vi "Build Dialog.vi"(8 "error in (no error)":errorcluster, 10 "Dialog VI":refnum<vi>, 11 "CS++Actor in":refnum<class "CS++Actor.lvclass">) -> (0 "error out":errorcluster, 3 "CS++Actor out":refnum<class "CS++Actor.lvclass">)   [LabVIEW 2015, in "CS++Actor.lvlib" / "CS++Actor.lvclass"]
uses:
  CS++Actor.lvclass
  <vilib>/Utility/traverseref.llb/TRef TravTarget.ctl
  <vilib>/Utility/VariantDataType/Type.ctl
  CS++Actor.lvclass/CS++Actor.ctl
  <vilib>/Utility/VariantDataType/VariantType.lvlib
  <vilib>/Utility/traverseref.llb/VI Scripting - Traverse.lvlib
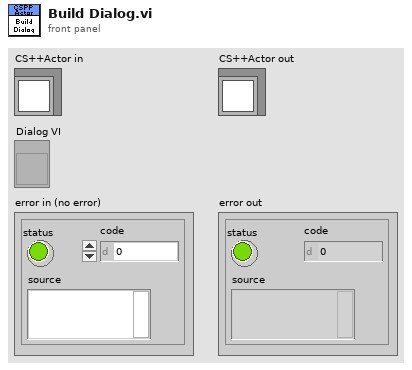
[diagram p1: front panel]
types:
  T1 = typedef "VariantType.lvlib/Type.ctl" = enum8{"Invalid Type", "Void", "I8", "I16", "I32", "I64", "U8", "U16", "U32", "U64", "Single Float", "Double Float", "Extended Float", "Single Complex", "Double Complex", "Extended Complex", "Enum U8", "Enum U16", "Enum U32", "Enum U64", "Single Float With Unit", "Double Float With Unit", "Extended Float With Unit", "Single Complex with Unit", "Double Complex with Unit", "Extended Complex with Unit", "Boolean", "String", "Path", "Picture", "Tag", "Array", "Cluster", "Variant", "LV Variant", "Waveform", "Timestamp", "Digital Waveform", "Digital Data", "ExpressData", "Refnum", "External Data", "VI", "Poly VI", "LabVIEW Class Instance", "Fixed Point"}
  T2 = typedef "TRef TravTarget.ctl" = enum16{"FP", "BD", "Other"}
  T3 = enum8{"Probe", "Diagram", "Panel Control", "3D Panel Control", "Dialog Panel Control", "Panel Indicator", "3D Panel Indicator", "Dialog Panel Indicator", "Power PC Control", "Power PC Indicator", "Silver Control", "Silver Indicator"}
  T4 = enum16{"Invalid Wire Rule", "Required", "Recommended", "Optional", "Dynamic Dispatch"}
  T5 = typedef "LVRectTypeDef.ctl" = cluster{"Left":i16, "Top":i16, "Right":i16, "Bottom":i16}
  T6 = enum16{"Invalid Wire Rule", "Required", "Recommended", "Optional", "Dynamic Dispatch"}[]
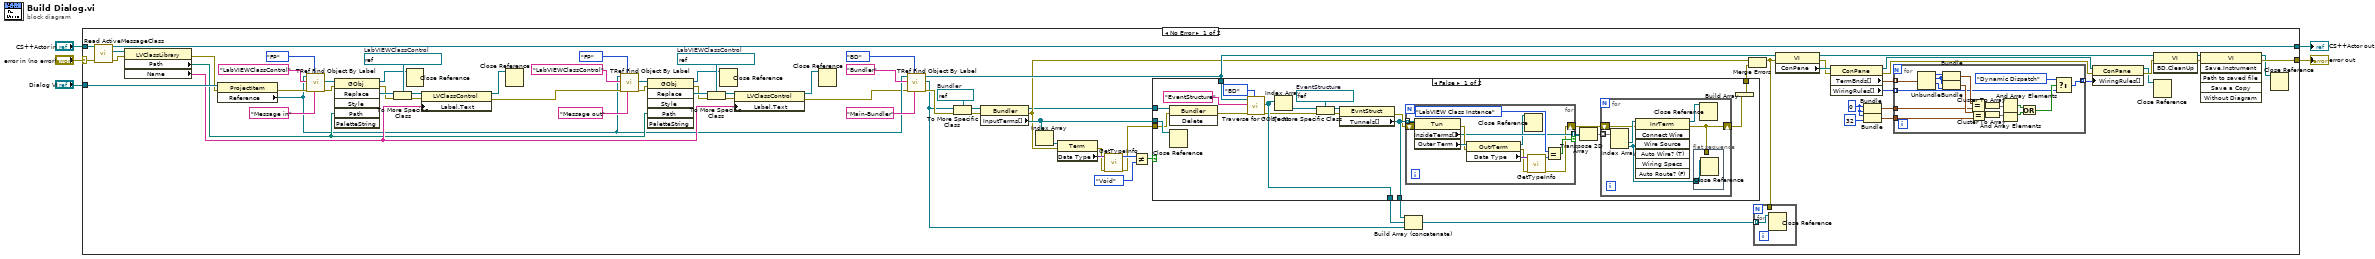
[diagram p0: block diagram]
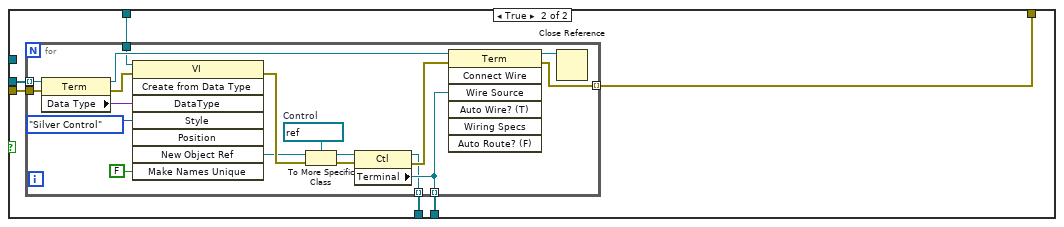
[diagram p2: hidden frame]
diagram:
  n1 = case shown="No Error" "error in (no error)" {
    selector: "error in (no error)" -> [w37 w168]
    tunnel: [w75 w168] -> w4
    tunnel: [w38 w167] -> w2
    tunnel: "CS++Actor in" -> [w39 w167]
    tunnel: "Dialog VI" -> [w84 _]
    frame No Error {
      w28 = refnum<vi> refnum  # LabVIEWClassControl
      w44 = refnum<vi> refnum  # LabVIEWClassControl
      w63 = i16 0
      w83 = refnum<vi> refnum  # Bundler
      n2 = call "Read ActiveMessageClass.vi"("error in (no error)"=w37, "CS++Actor in"=w39) -> ("error out"=w35:errorcluster, "ActiveMessageClass"=w36:refnum<vi>, "CS++Actor out"=w38:refnum<class "CS++Actor.lvclass">)  [unwired: 7 in]
      n3 = property class="LVClassLibrary"(reference=w36, error in=w35) -> (error out=w34:errorcluster, "Path"=w19:path, "Name"=w20:string)  [unwired: 1 out]
      n4 = property class="ProjectItem"(reference=w84, error in=w34) -> (error out=w49:errorcluster, "Reference"=w18:refnum<vi>)  [unwired: 1 out]
      n5 = call <vilib>:"TRef Find Object By Label.vi"("Label"="Message in", "Traverse Target"=TRef_TravTarget."FP", "error in (no error)"=w49, "Class Name"="LabVIEWClassControl", "VI Ref"=w18) -> ("error out"=w47:errorcluster, "Found Obj Ref"=w48:refnum<vi>)  [unwired: 3 in, 2 out]
      n6 = invoke class="GObj" method="Replace"(reference=w48, error in=w47, "Path"=w19) -> (reference out=w40:refnum<vi>, error out=w42:errorcluster, "Replace"=w43:refnum<vi>)  [unwired: 3 in, 3 out]
      n7 = To More Specific Class(target class=w44, reference=w43, error in=w42) -> (specific class reference=w46:refnum<vi>, error out=w45:errorcluster)
      n8 = Close Reference(reference=w40) -> ()  [unwired: 1 in, 1 out]
      n9 = property class="LVClassControl"(reference=w46, error in=w45, "Label.Text"=w20) -> (reference out=w41:refnum<vi>, error out=w21:errorcluster)
      n10 = Close Reference(reference=w41) -> ()  [unwired: 1 in, 1 out]
      n11 = call <vilib>:"TRef Find Object By Label.vi"("Label"="Message out", "Traverse Target"=TRef_TravTarget."FP", "error in (no error)"=w21, "Class Name"="LabVIEWClassControl", "VI Ref"=w18) -> ("error out"=w31:errorcluster, "Found Obj Ref"=w32:refnum<vi>)  [unwired: 3 in, 2 out]
      n12 = invoke class="GObj" method="Replace"(reference=w32, error in=w31, "Path"=w19) -> (reference out=w24:refnum<vi>, error out=w26:errorcluster, "Replace"=w27:refnum<vi>)  [unwired: 3 in, 3 out]
      n13 = To More Specific Class(target class=w28, reference=w27, error in=w26) -> (specific class reference=w30:refnum<vi>, error out=w29:errorcluster)
      n14 = Close Reference(reference=w24) -> ()  [unwired: 1 in, 1 out]
      n15 = property class="LVClassControl"(reference=w30, error in=w29, "Label.Text"=w20) -> (reference out=w25:refnum<vi>, error out=w17:errorcluster)
      n16 = Close Reference(reference=w25) -> ()  [unwired: 1 in, 1 out]
      n17 = call <vilib>:"TRef Find Object By Label.vi"("Label"="Main-Bundler", "Traverse Target"=TRef_TravTarget."BD", "error in (no error)"=w17, "Class Name"="Bundler", "VI Ref"=w18) -> ("error out"=w70:errorcluster, "Found Obj Ref"=w69:refnum<vi>, "dup VI Ref"=w68:refnum<vi>)  [unwired: 3 in, 1 out]
      n18 = To More Specific Class(target class=w83, reference=w69, error in=w70) -> (specific class reference=w82:refnum<vi>, error out=w81:errorcluster)
      n19 = property class="Bundler"(reference=w82, error in=w81) -> (reference out=w7:refnum<vi>, error out=w10:errorcluster, "InputTerms[]"=w15:refnum<vi>[])
      n20 = Index Array(array=w15) -> (element=w14:refnum<vi>)  [unwired: 1 in]
      n21 = property class="Term"(reference=w14, error in=w10) -> (error out=w6:errorcluster, "Data Type"=w13:variant)  [unwired: 1 out]
      n22 = call <vilib>:"GetTypeInfo.vi"("error in (no error)"=w6, "Variant"=w13) -> ("error out"=w9:errorcluster, "Type Enum"=w12:T1)  [unwired: 5 in, 3 out]
      n23 = Not Equal?(x=w12, y=Type."Void" ("Type Enum")) -> (x != y?=w8:bool)
      n24 = case shown="False" w8 {
        tunnel: [w91 w129] -> w80
        tunnel: [w97 w128] -> w79
        tunnel: w68 -> [w101 w127]
        tunnel: [w85 w126] -> w16
        tunnel: w15 -> [w104 w125]
        tunnel: w9 -> [w102 w124]
        tunnel: w7 -> [w103 _]
        frame False {
          w94 = refnum<vi> refnum  # EventStructure
          n25 = invoke class="Bundler" method="Delete"(reference=w103, error in=w102) -> (error out=w100:errorcluster)  [unwired: 1 in, 2 out]
          n26 = Close Reference(reference=w104) -> ()  [unwired: 1 in, 1 out]
          n27 = call <vilib>:"Traverse for GObjects.vi"("Traverse Target"=TRef_TravTarget."BD", "error in (no error)"=w100, "Class Name"="EventStructure", "VI Refnum"=w101) -> ("error out"=w96:errorcluster, "References"=w97:refnum<vi>[])  [unwired: 4 in, 2 out]
          n28 = Index Array(array=w97) -> (element=w95:refnum<vi>)  [unwired: 1 in]
          n29 = To More Specific Class(target class=w94, reference=w95, error in=w96) -> (specific class reference=w93:refnum<vi>, error out=w92:errorcluster)
          n30 = property class="EvntStruct"(reference=w93, error in=w92) -> (error out=w90:errorcluster, "Tunnels[]"=w91:refnum<vi>[])  [unwired: 1 out]
          n31 = for {
            tunnel: w91 -> [w123] mode=indexing
            tunnel: [w115] -> w89 mode=indexing if=w114
            shift-right: [w113] -> w87
            shift-left: w90 -> [w121]
            n32 = property class="Tun"(reference=w123, error in=w121) -> (error out=w117:errorcluster, "InsideTerms[]"=w115:refnum<vi>[], "Outer Term"=w122:refnum<vi>)  [unwired: 1 out]
            n33 = property class="OutrTerm"(reference=w122, error in=w117) -> (reference out=w112:refnum<vi>, error out=w116:errorcluster, "Data Type"=w120:variant)
            n34 = Close Reference(reference=w112) -> ()  [unwired: 1 in, 1 out]
            n35 = call <vilib>:"GetTypeInfo.vi"("error in (no error)"=w116, "Variant"=w120) -> ("error out"=w113:errorcluster, "Type Enum"=w119:T1)  [unwired: 5 in, 3 out]
            n36 = Equal?(x=Type."LabVIEW Class Instance" ("Type Enum"), y=w119) -> (x = y?=w114:bool)
          }
          n37 = Transpose 2D Array(2D array=w89) -> (transposed array=w88:refnum<vi>[][])
          n38 = for {
            tunnel: w88 -> [w110] mode=indexing
            shift-right: [w105] -> w86
            shift-left: w87 -> [w108]
            n39 = Index Array(array=w110) -> (element #1=w109:refnum<vi>, element #2=w106:refnum<vi>)  [unwired: 2 in]
            n40 = invoke class="InrTerm" method="Connect Wire"(reference=w109, error in=w108, "Wire Source"=w106) -> (reference out=w107:refnum<vi>, error out=w105:errorcluster)  [unwired: 4 in, 5 out]
            n41 = flat-sequence {
              tunnel: w106 -> [w111]
              tunnel: w105 -> [_]
              frame #0 {
                n42 = Close Reference(reference=w111) -> ()  [unwired: 1 in, 1 out]
              }
            }
            n43 = Close Reference(reference=w107) -> ()  [unwired: 1 in, 1 out]
          }
          n44 = Build Array(w86) -> (w85:errorcluster[])
        }
        frame True {
          n45 = for {
            tunnel: [w147] -> w126 mode=indexing
            tunnel: w125 -> [w144] mode=indexing
            tunnel: w124 -> [w143]
            tunnel: w127 -> [w140]
            tunnel: [w132] -> w129 mode=indexing
            tunnel: [w131] -> w128 mode=indexing
            w136 = refnum<vi> refnum  # Control
            n46 = property class="Term"(reference=w144, error in=w143) -> (reference out=w141:refnum<vi>, error out=w142:errorcluster, "Data Type"=w130:variant)
            n47 = invoke class="VI" method="Create from Data Type"(reference=w140, error in=w142, "DataType"=w130, "Style"=T3."Silver Control", "Make Names Unique"=FALSE ("Make Names Unique (F)")) -> (error out=w138:errorcluster, "New Object Ref"=w137:refnum<vi>)  [unwired: 3 in, 6 out]
            n48 = To More Specific Class(target class=w136, reference=w137, error in=w138) -> (specific class reference=w135:refnum<vi>, error out=w134:errorcluster)
            n49 = property class="Ctl"(reference=w135, error in=w134) -> (reference out=w131:refnum<vi>, error out=w133:errorcluster, "Terminal"=w132:refnum<vi>)
            n50 = invoke class="Term" method="Connect Wire"(reference=w141, error in=w133, "Wire Source"=w132) -> (reference out=w146:refnum<vi>, error out=w147:errorcluster)  [unwired: 4 in, 5 out]
            n51 = Close Reference(reference=w146) -> ()  [unwired: 1 in, 1 out]
          }
        }
      }
      n52 = Build Array (concatenate)(w80, w79, w69) -> (w78:refnum<vi>[])
      n53 = Merge Errors(w10, w16) -> (w66:errorcluster)
      n54 = for {
        tunnel: w78 -> [w166] mode=indexing
        tunnel: w66 -> [_]
        n55 = Close Reference(reference=w166) -> ()  [unwired: 1 in, 1 out]
      }
      n56 = property class="VI"(reference=w68, error in=w66) -> (reference out=w67:refnum<vi>, error out=w64:errorcluster, "ConPane"=w65:refnum<vi>)
      n57 = property class="ConPane"(reference=w65, error in=w64) -> (reference out=w56:refnum<vi>, error out=w54:errorcluster, "TermBnds[]"=w61:T5[], "WiringRules[]"=w58:T6)
      n58 = Bundle(w63, w63) -> (w60:cluster{i16, i16})  [unwired: 1 in]
      n59 = Bundle(w63, i16 32) -> (w59:cluster{i16, i16})  [unwired: 1 in]
      n60 = for {
        tunnel: w61 -> [w154] mode=indexing
        tunnel: w60 -> [w153]
        tunnel: w59 -> [w152]
        tunnel: w58 -> [w150] mode=indexing
        tunnel: [w148] -> w55 mode=indexing
        n61 = Unbundle(w154) -> ("Left"=w165:i16, "Top"=w155:i16, "Right"=w156:i16)  [unwired: 1 out]
        n62 = Bundle("Left"=w165, "Top"=w155) -> (w164:cluster{"Left":i16, "Top":i16})  [unwired: 1 in]
        n63 = Bundle("Top"=w155, "Right"=w156) -> (w163:cluster{"Top":i16, "Right":i16})  [unwired: 1 in]
        n64 = Equal?(x=w164, y=w153) -> (x = y?=w162:cluster{bool, bool})
        n65 = Equal?(x=w163, y=w152) -> (x = y?=w161:cluster{bool, bool})
        n66 = Cluster To Array(cluster=w162) -> (array=w160:bool[])
        n67 = Cluster To Array(cluster=w161) -> (array=w159:bool[])
        n68 = And Array Elements(Boolean array=w160) -> (logical AND=w158:bool)
        n69 = And Array Elements(Boolean array=w159) -> (logical AND=w157:bool)
        n70 = Or(x=w158, y=w157) -> (x .or. y?=w151:bool)
        n71 = Select(t=T4."Dynamic Dispatch" ("Wire Rule"), s=w151, f=w150) -> (s? t:f=w148:T4)
      }
      n72 = property class="ConPane"(reference=w56, error in=w54, "WiringRules[]"=w55) -> (reference out=w53:refnum<vi>, error out=w57:errorcluster)
      n73 = invoke class="VI" method="BD.CleanUp"(reference=w67, error in=w57) -> (reference out=w77:refnum<vi>, error out=w76:errorcluster)  [unwired: 1 in, 1 out]
      n74 = Close Reference(reference=w53) -> ()  [unwired: 1 in, 1 out]
      n75 = invoke class="VI" method="Save.Instrument"(reference=w77, error in=w76) -> (reference out=w74:refnum<vi>, error out=w75:errorcluster)  [unwired: 4 in, 4 out]
      n76 = Close Reference(reference=w74) -> ()  [unwired: 1 in, 1 out]
    }
    frame Error {
    }
  }
  "error out" <- w4
  "CS++Actor out" <- w2
